vi "LVCAM Nest Destroyed.vi"(9 "Nest Error":errorcluster, 10 "Nest Actor":refnum<class "Actor.lvclass">, 11 "Actor in":refnum<class "Self Actor.lvclass">) -> (0 "error out":errorcluster, 3 "Actor out":refnum<class "Self Actor.lvclass">)   [LabVIEW 2021, in "LVCAM.lvlib" / "Self Actor.lvclass"]
uses:
  Self Actor.lvclass
  C:/PPLs/LabVIEW-Composed-Actor-Model-LVCAM/LabVIEW-Composed-Actor-Model-LVCAM/LVCAM/LVCAM/Actor/Actor.lvclass
  Actor/Actor.lvclass
  Self Actor.lvclass/Self Actor.ctl
  Msgs/LVCAM Destroy Self/LVCAM Destroy Self Msg/LVCAM Destroy Self Msg.lvclass
  C:/PPLs/LabVIEW-Composed-Actor-Model-LVCAM/LabVIEW-Composed-Actor-Model-LVCAM/LVCAM/LVCAM/Msg Strategy/Msg Strategy.lvclass
  Self Msg Send.vi
  LVCAM.lvlib
  C:/PPLs/LabVIEW-Composed-Actor-Model-LVCAM/LabVIEW-Composed-Actor-Model-LVCAM/LVCAM/Msgs/Actor Create/Actor Create/Actor Create.lvclass
  C:/PPLs/LabVIEW-Composed-Actor-Model-LVCAM/LabVIEW-Composed-Actor-Model-LVCAM/LVCAM/Msgs/LVCAM Destroy Self/LVCAM Destroy Self/LVCAM Destroy Self.lvclass
  C:/PPLs/LabVIEW-Composed-Actor-Model-LVCAM/LabVIEW-Composed-Actor-Model-LVCAM/LVCAM/Msgs/LVCAM Nest Destroyed/LVCAM Nest Destroyed/LVCAM Nest Destroyed.lvclass
  C:/PPLs/LabVIEW-Composed-Actor-Model-LVCAM/LabVIEW-Composed-Actor-Model-LVCAM/LVCAM/LVCAM/Self Actor/Self Actor.lvclass
  C:/PPLs/LabVIEW-Composed-Actor-Model-LVCAM/LabVIEW-Composed-Actor-Model-LVCAM/LVCAM/Msgs/LVCAM Destroy Self/LVCAM Destroy Self Msg/LVCAM Destroy Self Msg.lvclass
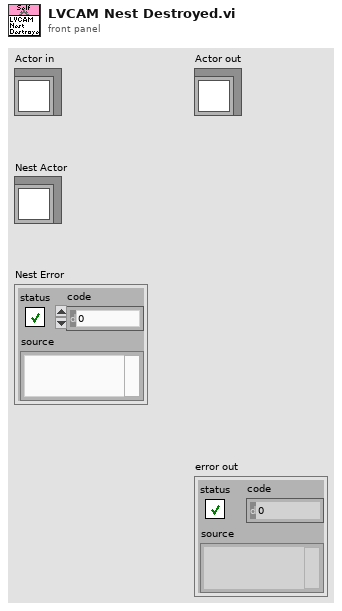
[diagram p1: front panel]
types:
  T1 = typedef "LVCAM.lvlib/Self Actor.lvclass/State.ctl" = enum16{"Msging", "Destroying"}
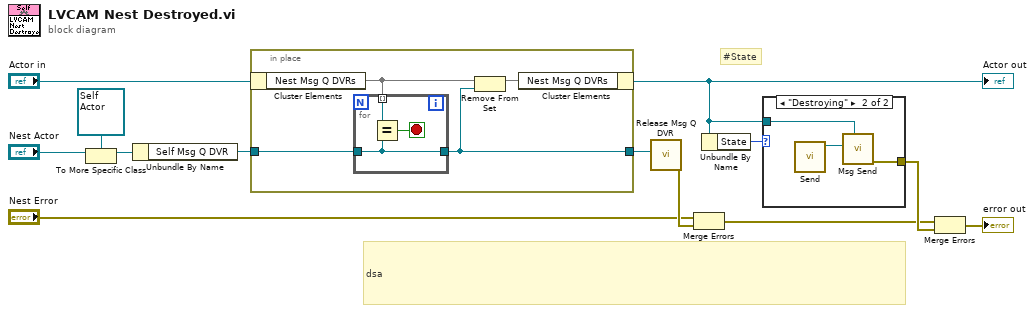
[diagram p0: block diagram]
diagram:
  # "dsa"
  # "#State"
  n1 = To More Specific Class(target class=refnum<class "Self Actor.lvclass"> refnum ("Artifex Actor Model.lvlib:Self Actor.lvclass"), reference="Nest Actor") -> (specific class reference=w13:refnum<class "Self Actor.lvclass">)  [unwired: 1 in, 1 out]
  n2 = Unbundle By Name(w13) -> ("Self Msg Q DVR"=w6:refnum<data-value>)
  n3 = in-place {
    in-place-border: w6 -> [w15]
    in-place-border: [w14] -> w5
    n4 = in-place-cluster #1("Actor in") -> ("Nest Msg Q DVRs"=w17:set{refnum<data-value>})
    n5 = for {
      tunnel: w15 -> [w18]
      tunnel: w17 -> [w19] mode=indexing
      tunnel: [w18] -> w14
      stop <- w20 stop-if-true
      n6 = Equal?(x=w19, y=w18) -> (x = y?=w20:bool)
    }
    n7 = Remove From Set(10:w14, 11:w17) -> (3:w16:set{refnum<data-value>})  [unwired: 1 out]
    n8 = in-place-cluster #1("Nest Msg Q DVRs"=w16) -> (w1:refnum<class "Self Actor.lvclass">)
  }
  "Actor out" <- w1
  n9 = call "Release Msg Q DVR.vi"("Msg Q DVR"=w5) -> ("error out"=w3:errorcluster)  [unwired: 10 in]
  n10 = Merge Errors("Nest Error", w3) -> (w4:errorcluster)
  n11 = Unbundle By Name(w1) -> ("State"=w9:T1)
  n12 = case shown="\"Destroying\"" w9 {
    tunnel: w1 -> [_ w22]
    tunnel: [_ w21] -> w7
    frame "Msging" {
    }
    frame "Destroying" {
      n13 = call "Send.vi"() -> ("LVCAM Destroy Self Msg out"=w23:refnum<class "LVCAM Destroy Self Msg.lvclass">)  [unwired: 11 in]
      n14 = call-poly "Msg Send.vi"("Actor"=w22, "Msg"=w23) -> ("error out"=w21:errorcluster)  [unwired: 9 in]
    }
  }
  n15 = Merge Errors(w4, w7) -> (→"error out":errorcluster)
